vi "3 Wheels.vi"() -> ()   [LabVIEW 2019, in "3_Wheels.xctl"]
uses:
  3_Wheels.xctl
  <vilib>/vision/Image Controls.llb/IMAQ Image.ctl
panel:
  in  "Cluster":T2={"InCluster"={"MotorSpeed0"=0.0, "MotorSpeed1"=0.0, "MotorSpeed2"=0.0, "MotorSpeed3"=0.0, "HCDIO 1"=0.0, "HCDIO 2"=0.0, "HCDIO 3"=0.0, "HCDIO 4"=0.0, "HCDIO 5"=0.0, "HCDIO 6"=0.0, "HCDIO 7"=0.0, "HCDIO 8"=0.0, "HCDIO 9"=0.0, "HCDIO 10"=0.0}, "In_Cluster"={"MotorEnc0"=0.0, "MotorEnc1"=0.0, "MotorEnc2"=0.0, "MotorEnc3"=0.0, "US1"=0.0, "US2"=0.0, "Analog1"=0.0, "Analog2"=0.0, "Analog3"=0.0, "Analog4"=0.0, "IMU"=0.0, "TitanLimits"=[FALSE, FALSE, FALSE, FALSE, FALSE, FALSE, FALSE, FALSE], "Flexs"=[FALSE, FALSE, FALSE, FALSE, FALSE, FALSE, FALSE, FALSE], "Camera"="RobocadImage"}}
  out "Enc_2":dbl
  out "Enc_1":dbl
  out "Enc_0":dbl
  out "Motor_2":dbl
  out "Motor_1":dbl
  out "Motor_0":dbl
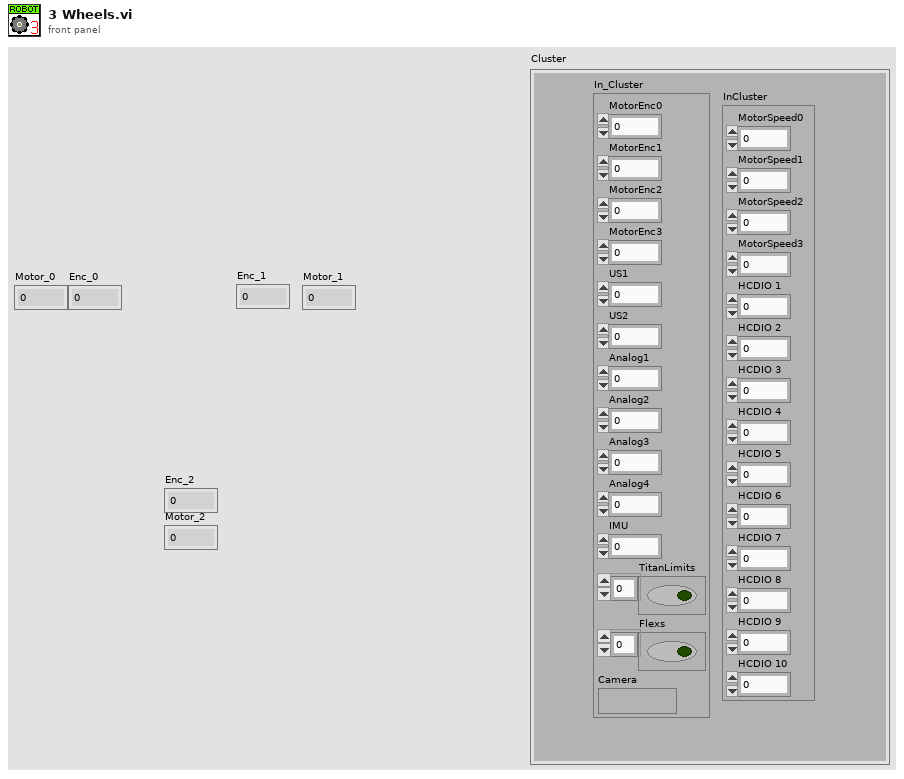
[diagram p1: front panel]
types:
  T1 = typedef "IMAQ Image.ctl" = refnum<image>
  T2 = cluster{"InCluster":cluster{"MotorSpeed0":dbl, "MotorSpeed1":dbl, "MotorSpeed2":dbl, "MotorSpeed3":dbl, "HCDIO 1":dbl, "HCDIO 2":dbl, "HCDIO 3":dbl, "HCDIO 4":dbl, "HCDIO 5":dbl, "HCDIO 6":dbl, "HCDIO 7":dbl, "HCDIO 8":dbl, "HCDIO 9":dbl, "HCDIO 10":dbl}, "In_Cluster":cluster{"MotorEnc0":dbl, "MotorEnc1":dbl, "MotorEnc2":dbl, "MotorEnc3":dbl, "US1":dbl, "US2":dbl, "Analog1":dbl, "Analog2":dbl, "Analog3":dbl, "Analog4":dbl, "IMU":dbl, "TitanLimits":bool[], "Flexs":bool[], "Camera":T1}}
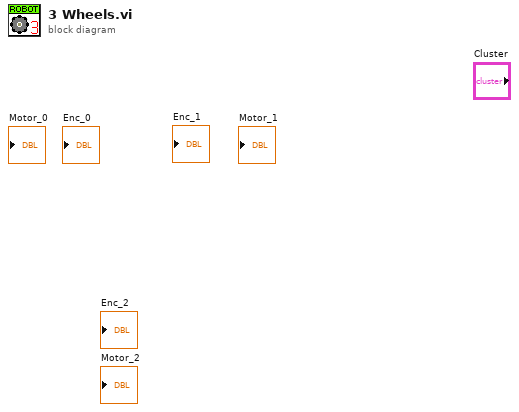
[diagram p0: block diagram]
diagram:
